vi "Servo Demo.vi"() -> ()   [LabVIEW 2023, in "CTI-Visa-Scratchpad.lvlib"]
uses:
  CTI-Visa-Scratchpad.lvlib
  CTI-Visa/CTI-Visa.lvlib
panel:
  out "Freq Hz":sgl
  out "Duty % (0-1)":sgl
  in  "GPIO":i32
  in  "stop":bool
  in  "Angle":dbl(slide)=90.0 scale=0.0..180.0
  in  "Port":refnum<visa-resource-name>="COM3"
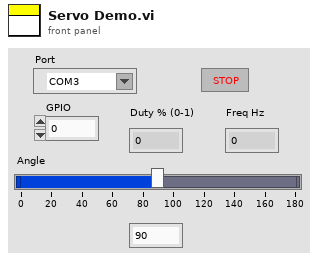
[diagram p1: front panel]
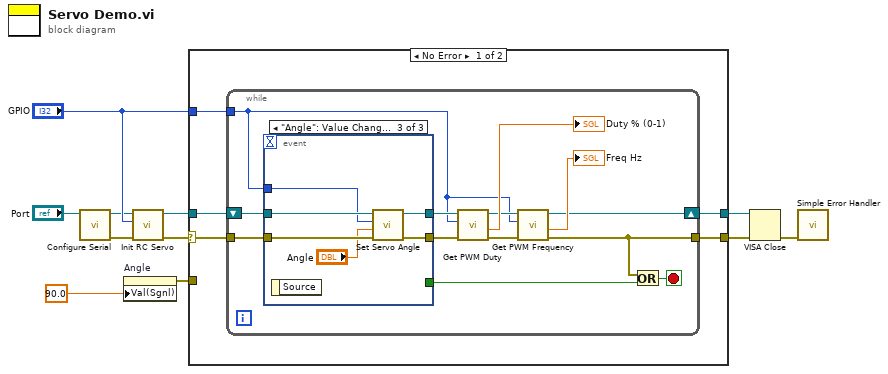
[diagram p0: block diagram]
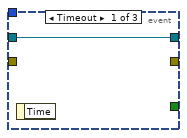
[diagram p2: hidden frame]
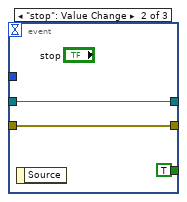
[diagram p3: hidden frame]
diagram:
  n1 = call "Configure Serial.vi"("VISA resource name in"="Port") -> ("error out"=w1:errorcluster, "VISA resource name"=w2:refnum<visa-resource-name>)  [unwired: 9 in]
  n2 = property on="Angle" class="Slide (strict)"("Val(Sgnl)"=90.0 ("Value (Signaling)")) -> (error out=w4:errorcluster)  [unwired: 2 in, 1 out]
  n3 = call "Init RC Servo.vi"("error in (no error)"=w1, "GPIO"="GPIO", "VISA resource name in"=w2) -> ("error out"=w10:errorcluster, "VISA resource name"=w11:refnum<visa-resource-name>)  [unwired: 7 in]
  n4 = case shown="No Error" w10 {
    selector: w10 -> [w15 w41]
    tunnel: w11 -> [w16 w40]
    tunnel: [w13 w41] -> w8
    tunnel: [w14 w40] -> w9
    tunnel: "GPIO" -> [w12 _]
    tunnel: w4 -> [_ _]
    frame No Error {
      n5 = while {
        shift-right: [w18] -> w14
        shift-left: w16 -> [w28]
        tunnel: w15 -> [w27]
        tunnel: [w17] -> w13
        tunnel: w12 -> [w20]
        stop <- w26 stop-if-true
        n6 = event shown="[2] \"Angle\": Value Change" {
          selector: _ -> [_ _ _]
          dyn-events: _ -> [_ _ _]
          timeout: _ -> [_ _ _]
          tunnel: [_ TRUE _] -> w29
          tunnel: [w30 w32 w36] -> w25
          tunnel: w28 -> [w30 w32 w39]
          tunnel: w27 -> [_ w31 w38]
          tunnel: [_ w31 w37] -> w24
          tunnel: w20 -> [_ _ w34]
          event Timeout {
            n7 = event-data() -> ()  [unwired: 1 in, 1 out]
          }
          event "stop": Value Change {
            n8 = event-data() -> ()  [unwired: 1 in, 1 out]
          }
          event "Angle": Value Change {
            n9 = event-data() -> ()  [unwired: 1 in, 1 out]
            n10 = call "Set Servo Angle.vi"("error in (no error)"=w38, "Angle (0 - 180)"="Angle", "GPIO"=w34, "VISA resource name in"=w39) -> ("error out"=w37:errorcluster, "VISA resource name"=w36:refnum<visa-resource-name>)  [unwired: 6 in]
          }
        }
        n11 = call "Get PWM Duty.vi"("error in (no error)"=w24, "Channel"=w20, "VISA resource name in"=w25) -> ("error out"=w21:errorcluster, "Duty % (0-1)"=→"Duty % (0-1)":sgl, "VISA resource name"=w22:refnum<visa-resource-name>)  [unwired: 6 in]
        n12 = call "Get PWM Frequency.vi"("error in (no error)"=w21, "Channel"=w20, "VISA resource name in"=w22) -> ("error out"=w17:errorcluster, "Freq Hz"=→"Freq Hz":sgl, "VISA resource name"=w18:refnum<visa-resource-name>)  [unwired: 6 in]
        n13 = Or(x=w17, y=w29) -> (x .or. y?=w26:bool)
      }
    }
    frame Error {
    }
  }
  n14 = VISA Close(VISA resource name=w9, error in (no error)=w8) -> (error out=w7:errorcluster)
  n15 = call <vilib>:"Simple Error Handler.vi"("error in (no error)"=w7) -> ()  [unwired: 4 in, 5 out]
